vi "WPI_SwitchOpenCounting.vi"(7 "Normally Closed":bool, 8 "error in (no error)":errorcluster, 9 "Filter Frequency (Hz)":dbl=60.0 format="%#_13g", 10 "DIO Channel":T1) -> (0 "error out":errorcluster, 3 "SwitchDevRef":T2={"DevStatus"={"status"=FALSE, "code"=0, "source"=""}, "DIO Channel"=enum."Invalid", "CntIndex"=enum."Invalid", "Normally Closed"=FALSE})   [LabVIEW 2017]
doc: "Creates a reference to the switch you specify. You must open a reference before using any other VIs on this palette.\n\nThis software is licensed. Open the labview\\readme\\WPI Robotics Library Open Source License.txt file for more information."
uses:
  <vilib>/Rock Robotics/WPI/Switch/WPI_SwitchDevRef.ctl
  <vilib>/Rock Robotics/SystemInterfaces/DIO/FPGA_DIOChannel.ctl
  <vilib>/Rock Robotics/SystemInterfaces/Counter/FPGA_CounterCtrSystemIndex.ctl
  <vilib>/Rock Robotics/WPI/Counter/WPI_CounterDigitalInputToDigitalSource.vi
  <vilib>/Rock Robotics/WPI/Counter/WPI_CounterOpen UpDown Mode.vi
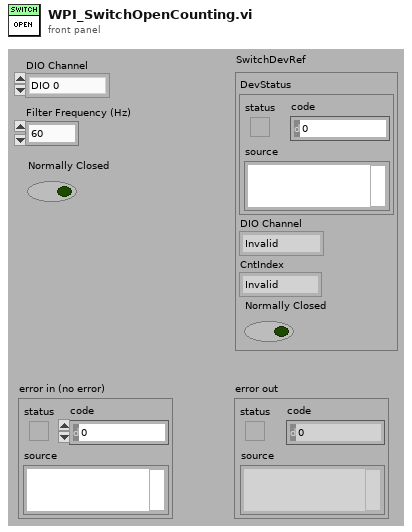
[diagram p1: front panel]
types:
  T1 = typedef "FPGA_DIOChannel.ctl" = enum8{"DIO 0", "DIO 1", "DIO 2", "DIO 3", "DIO 4", "DIO 5", "DIO 6", "DIO 7", "DIO 8", "DIO 9", "DIO MXP 0", "DIO MXP 1", "DIO MXP 2", "DIO MXP 3", "DIO MXP 4", "DIO MXP 5", "DIO MXP 6", "DIO MXP 7", "DIO MXP 8", "DIO MXP 9", "DIO MXP 10", "DIO MXP 11", "DIO MXP 12", "DIO MXP 13", "DIO MXP 14", "DIO MXP 15", "SPI Port CS1", "SPI Port CS2", "SPI Port CS3", "SPI Port MISO", "SPI Port MOSI", "Invalid"}
  T2 = typedef "WPI_SwitchDevRef.ctl" = cluster{"DevStatus":errorcluster, "DIO Channel":T1, "CntIndex":T3, "Normally Closed":bool}
  T3 = typedef "FPGA_CounterCtrSystemIndex.ctl" = enum8{"Ctr 0", "Ctr 1", "Ctr 2", "Ctr 3", "Ctr 4", "Ctr 5", "Ctr 6", "Ctr 7", "Invalid"}
  T4 = enum16{"Rising Edge", "Falling Edge", "Raising & Falling Edge", "Disabled"}
  T5 = typedef "WPI_DigitalInputDevRef.ctl" = cluster{"DevStatus":errorcluster, "DIO Channel":T1}
  T6 = typedef "FPGA_CounterEncoderSourceConvertionLVSourceType.ctl" = cluster{"DevStatus":errorcluster, "AnalogTriggerMode?":bool, "DigitalMode":cluster{"DIO Channel":T7}, "AnalogTriggerMode":cluster{"AnalogTriggerIndex":T8, "OutputType":T9}}
  T7 = typedef "FPGA_DIODigitalSourceChannel.ctl" = enum8{"DIO 0", "DIO 1", "DIO 2", "DIO 3", "DIO 4", "DIO 5", "DIO 6", "DIO 7", "DIO 8", "DIO 9", "DIO MXP 0", "DIO MXP 1", "DIO MXP 2", "DIO MXP 3", "DIO MXP 4", "DIO MXP 5", "DIO MXP 6", "DIO MXP 7", "DIO MXP 8", "DIO MXP 9", "DIO MXP 10", "DIO MXP 11", "DIO MXP 12", "DIO MXP 13", "DIO MXP 14", "DIO MXP 15", "Disabled"}
  T8 = typedef "FPGA_AnalogTriggerIndex.ctl" = enum8{"Trig 0", "Trig 1", "Trig 2", "Trig 3", "Trig 4", "Trig 5", "Trig 6", "Trig 7", "Invalid"}
  T9 = typedef "FPGA_AnalogTriggerOutType.ctl" = enum16{"InWindow", "TriggerState", "Rising", "Falling"}
  T10 = typedef "WPI_CounterDevRef.ctl" = cluster{"DevStatus":errorcluster, "CntIndex":T3}
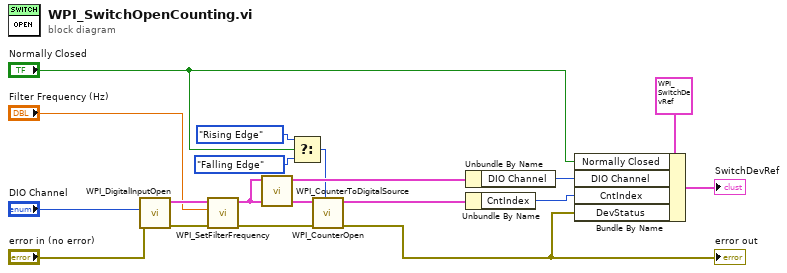
[diagram p0: block diagram]
diagram:
  n1 = call <vilib>:"WPI_DigitalInputOpen.vi"("error in (no error)"="error in (no error)", "DIO Channel"="DIO Channel") -> ("error out"=w13:errorcluster, "DigitalInputDevRef"=w12:T5)  [unwired: 8 in]
  n2 = call <vilib>:"WPI_SetFilterFrequency.vi"("error in (no error)"=w13, "Filter Frequency"="Filter Frequency (Hz)", "DigitalInputDevRef"=w12) -> ("error out"=w9:errorcluster, "DigitalInputDevRef"=w7:T5)  [unwired: 7 in]
  n3 = call-poly <vilib>:"WPI_CounterToDigitalSource.vi"("DigitalInputDevRef"=w7) -> ("Digital Source"=w10:T6)  [unwired: 6 out]
  n4 = Select(t=T4."Rising Edge" ("UpEdge"), s="Normally Closed", f=T4."Falling Edge" ("UpEdge")) -> (s? t:f=w4:T4)
  n5 = call-poly <vilib>:"WPI_CounterOpen.vi"("UpEdge"=w4, "error in (no error)"=w9, "Up Source"=w10) -> ("error out"=w1:errorcluster, "CounterDevRef"=w2:T10)  [unwired: 4 in, 3 out]
  "error out" <- w1
  n6 = Unbundle By Name(w7) -> ("DIO Channel"=w14:T1)
  n7 = Unbundle By Name(w2) -> ("CntIndex"=w8:T3)
  n8 = Bundle By Name(cluster=T2 {"DevStatus"={"status"=FALSE, "code"=0, "source"=""}, "DIO Channel"=enum."Invalid", "CntIndex"=enum."Invalid", "Normally Closed"=FALSE} ("SwitchDevRef"), "Normally Closed"="Normally Closed", "DIO Channel"=w14, "CntIndex"=w8, "DevStatus"=w1) -> (→"SwitchDevRef":T2)
